vi "NI PID Comparison 2.vi"() -> ()   [LabVIEW 2015]
doc: "This example demonstrates how to simulate a general PID controller."
uses:
  library/Gains.ctl
  library/Anti-Windup Method.ctl
  library/Output Range.ctl
  <vilib>/addons/control/pid/pid.llb/PID Structure.ctl
  <vilib>/addons/control/pid/pid.llb/PID Time Unit.ctl
  <vilib>/addons/control/pid/pid.llb/PID Structure Conversion (DBL).vi
  <vilib>/addons/control/pid/pid.llb/PID (DBL).vi
  <vilib>/addons/control/pid/NI_PID_pid.lvlib
  library/PID.lvlib
panel:
  in  "Back-Calculation Gain Kb":dbl format="%#_13g"
  in  "Anti-Windup Method":T1
  in  "Gains":T2={"Kp"=20.0, "Ki"=0.05, "Kd"=0.0}
  out "Process Variable and Setpoint":cluster{"initial PV":dbl, "SP:":dbl}(graph)
  out "PV":dbl(slide)=60.754431603254424 scale=0.0..100.0
  out "MV":dbl(slide)=18.78965245852964 scale=-100.0..100.0
  out "Manipulated Variable":dbl(graph)
  out "NI PID Manipulated Variable":dbl(graph)
  in  "SP:":dbl(slide)=43.790849673202615 min=0.0 max=0.0 scale=0.0..100.0
  out "MV:":dbl(slide)=18.78965245852964 scale=-100.0..100.0
  out "PV:":dbl(slide)=60.754431603254424 scale=0.0..100.0
  in  "Stop":bool
  out "NI PID Process Variable and Setpoint":cluster{"initial PV":dbl, "SP:":dbl}(graph)
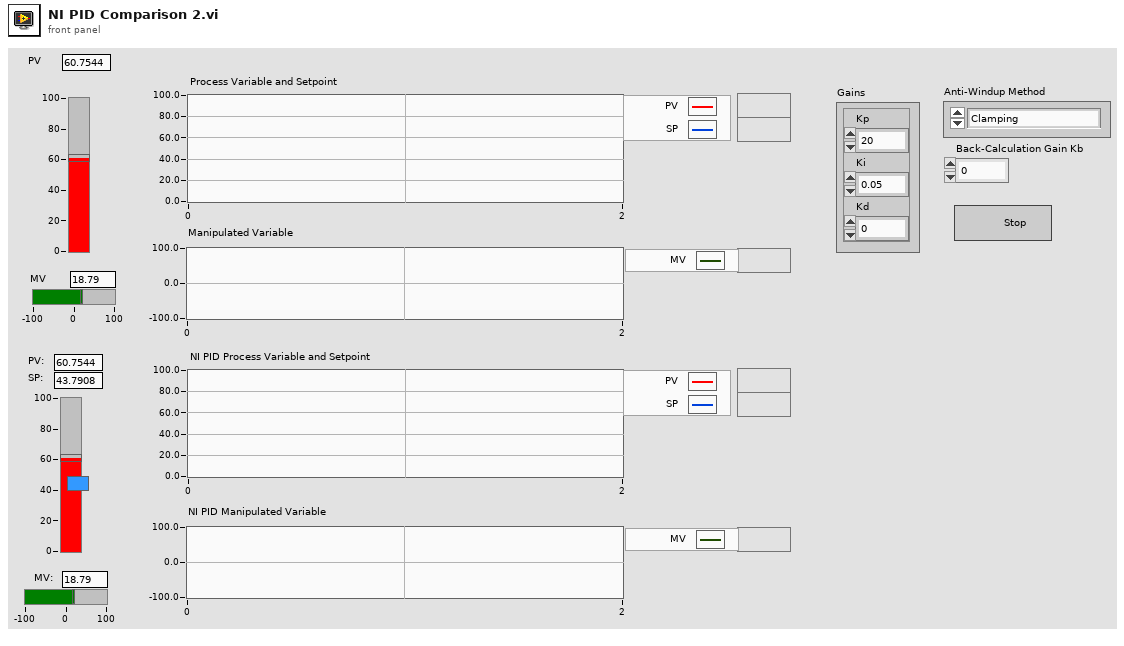
[diagram p1: front panel]
types:
  T1 = typedef "PID.lvlib/Anti-Windup Method.ctl" = enum16{"Clamping", "Back-Calculation", "None"}
  T2 = typedef "PID.lvlib/Gains.ctl" = cluster{"Kp":dbl, "Ki":dbl, "Kd":dbl}
  T3 = typedef "PID.lvlib/Output Range.ctl" = cluster{"Output Min":dbl, "Output Max":dbl}
  T4 = typedef "PID.lvlib/PID.ctl" = cluster{"Accumulated Error":dbl, "Kb":dbl, "Anti-Windup Method":T1, "Previous Error":dbl, "Gains":T2, "Output Range":T3}
  T5 = typedef "NI_PID_pid.lvlib/PID Time Unit.ctl" = u16
  T6 = typedef "NI_PID_pid.lvlib/PID Structure.ctl" = u16
  T7 = cluster{"static gain":dbl, "lag (min)":dbl, "dead cycles":dbl, "load %":dbl, "deadband":dbl, "noise level %":dbl, "initial PV":dbl, "initial PV 2":dbl}
  T8 = cluster{"proportional gain (Kc)":dbl, "integral time (Ti, min)":dbl, "derivative time (Td, min)":dbl}
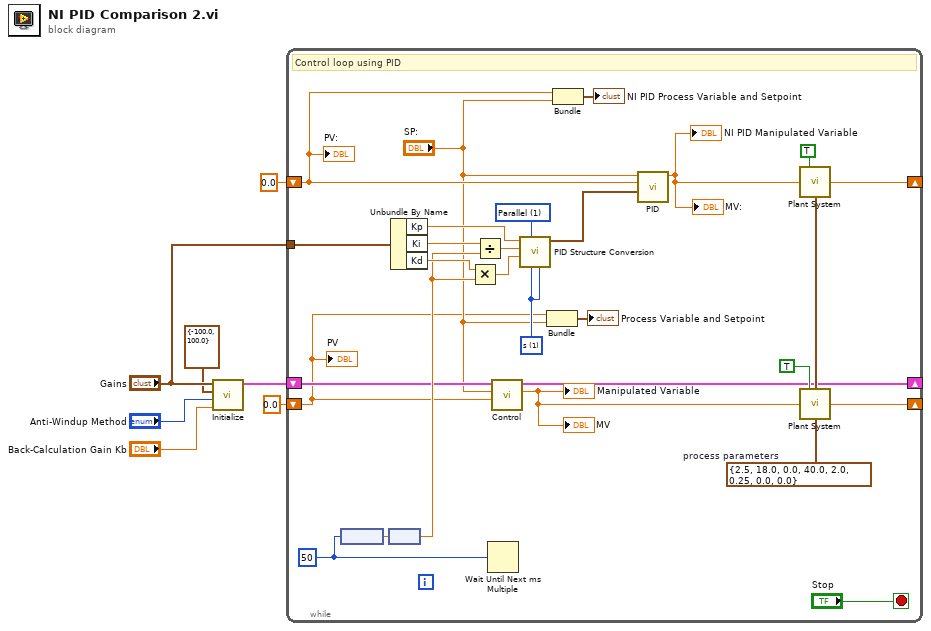
[diagram p0: block diagram]
diagram:
  n1 = call "Initialize.vi"("Back-Calculation Gain Kb (1)"="Back-Calculation Gain Kb", "Anti-Windup Method (Clamping)"="Anti-Windup Method", "Output Range"=T3 {"Output Min"=-100.0, "Output Max"=100.0}, "Gains"="Gains") -> ("PID"=w1:T4)  [unwired: 7 in]
  n2 = while {
    shift-left: 0.0 ("Plant Output") -> [w32]
    shift-right: [w33] -> _
    shift-right: [w28] -> _
    shift-left: 0.0 ("Plant Output") -> [w8]
    tunnel: "Gains" -> [w13]
    shift-right: [w11] -> _
    shift-left: w1 -> [w12]
    stop <- "Stop" stop-if-true
    w15 = T5 1 items=["min", "s"] ("integral unit")
    w26 = T6 1 items=["Academic (Standard)", "Parallel", "Series"] ("PID structure")
    w24 = T7 {"static gain"=2.5, "lag (min)"=18.0, "dead cycles"=0.0, "load %"=40.0, "deadband"=2.0, "noise level %"=0.25, "initial PV"=0.0, "initial PV 2"=0.0}  # process parameters
    w23 = u32 50 ("unsigned 32bit integer")
    # "Control loop using PID"
    n3 = node(w23) -> (w22:dbl[unit])
    n4 = node(w22) -> (w16:dbl)
    n5 = Unbundle By Name(w13) -> ("Kp"=w21:dbl, "Ki"=w17:dbl, "Kd"=w19:dbl)
    n6 = Multiply(x=w19, y=w16) -> (x*y=w20:dbl)
    n7 = Divide(x=w17, y=w16) -> (x/y=w18:dbl)
    n8 = Wait Until Next ms Multiple(millisecond multiple=w23) -> ()  [unwired: 1 out]
    n9 = call "Control.vi"("Process Variable"=w8, "Setpoint"="SP:", "PI-Controller in"=w12) -> ("Output"=w10:dbl, "PID out"=w11:T4)  [unwired: 7 in]
    "MV" <- w10
    "Manipulated Variable" <- w10
    n10 = call-poly <vilib>:"PID Structure Conversion.vi"("derivative unit"=w15, "integral unit"=w15, "PID structure"=w26, "derivative"=w20, "integral"=w18, "proportional"=w21) -> ("PID gains"=w25:T8)  [unwired: 5 in]
    n11 = Bundle("Plant Output"=w8, "SP:"="SP:") -> (→"Process Variable and Setpoint":cluster{"Plant Output":dbl, "SP:":dbl})  [unwired: 1 in]
    n12 = Bundle("Plant Output"=w32, "SP:"="SP:") -> (→"NI PID Process Variable and Setpoint":cluster{"Plant Output":dbl, "SP:":dbl})  [unwired: 1 in]
    n13 = call-poly <vilib>:"PID.vi"("PID gains"=w25, "process variable"=w32, "setpoint"="SP:") -> ("output"=w30:dbl)  [unwired: 7 in, 1 out]
    "MV:" <- w30
    "NI PID Manipulated Variable" <- w30
    n14 = call "Plant System.vi"("Integrator ?"=TRUE, "Plant Input"=w30, "process parameters"=w24) -> ("Plant Output"=w33:dbl)  [unwired: 12 in]
    n15 = call "Plant System.vi"("Integrator ?"=TRUE, "Plant Input"=w10, "process parameters"=w24) -> ("Plant Output"=w28:dbl)  [unwired: 12 in]
    "PV:" <- w32
    "PV" <- w8
  }
